vi "test_F9P_fgv-ver.vi"() -> ()   [LabVIEW 2019] (continued)
357,28,09,08,194,,1*72\r\n$GBGSV,5,3,17,10,14,222,31,11,34,144,33,13,50,316,32,14,73,036,27,1*77\r\n$GBGSV,5,4,17,16,25,186,,27,10,317,,28,61,308,30,33,75,244,42,1*7C\r\n$GBGSV,5,5,17,34,11,143,22,1*41\r\n$GBGSV,5,1,17,01,42,153,,03,45,207,,04,35,133,,05,09,257,,3*7E\r\n$GBGSV,5,2,17,06,29,183,,07,08,201,,08,66,357,16,09,08,194,,3*7D\r\n$GBGSV,5,3,17,10,14,222,32,11,34,144,46,13,50,316,21,14,73,036,27,3*76\r\n$GBGSV,5,4,17,16,25,186,36,27,10,317,,28,61,308,,33,75,244,,3*7E\r\n$GBGSV,5,5,17,34,11,143,,3*43\r\n$GNGLL,3723.57124,N,12657.01326,E,064943.00,A,A*7A\r\n$GNRMC,064944.00,A,3723.57121,N,12657.01327,E,0.019,,250720,,,A,V*10\r\n$GNVTG,,T,,M,0.019,N,0.036,K,A*30\r\n$GNGGA,064944.00,3723.57121,N,12657.01327,E,1,12,0.74,36.2,M,18.5,M,,*77\r\n$GNGSA,A,3,17,19,06,12,05,02,09,,,,,,1.35,0.74,1.12,1*02\r\n$GNGSA,A,3,85,70,71,72,,,,,,,,,1.35,0.74,1.12,2*0D\r\n$GNGSA,A,3,36,11,04,09,12,,,,,,,,1.35,0.74,1.12,3*0E\r\n$GNGSA,A,3,28,11,14,13,33,08,34,10,,,,,1.35,0.74,1.12,4*01\r\n$GPGSV,4,1,13,02,67,338,32,04,06,036,21,05,50,265,44,06,56,081,46,1*62\r\n$GPGSV,4,2,13,07,08,102,19,09,36,055,39,12,17,260,32,13,11,191,31,1*6B\r\n$GPGSV,4,3,13,17,16,158,42,19,34,162,41,25,11,291,25,29,09,322,35,1*68\r\n$GPGSV,4,4,13,30,03,132,,1*56\r\n$GPGSV,4,1,13,02,67,338,,04,06,036,,05,50,265,35,06,56,081,33,6*63\r\n$GPGSV,4,2,13,07,08,102,,09,36,055,22,12,17,260,30,13,11,191,,6*6E\r\n$GPGSV,4,3,13,17,16,158,35,19,34,162,,25,11,291,22,29,09,322,13,6*69\r\n$GPGSV,4,4,13,30,03,132,,6*51\r\n$GLGSV,2,1,06,70,51,030,19,71,72,230,44,72,20,218,35,84,06,136,08,1*7B\r\n$GLGSV,2,2,06,85,61,118,44,86,55,338,,1*7A\r\n$GLGSV,2,1,06,70,51,030,,71,72,230,28,72,20,218,36,84,06,136,13,3*72\r\n$GLGSV,2,2,06,85,61,118,33,86,55,338,,3*78\r\n$GAGSV,3,1,09,02,03,285,07,04,67,079,38,05,00,212,,09,47,197,33,7*70\r\n$GAGSV,3,2,09,11,78,050,29,12,30,117,32,18,58,277,45,19,15,041,08,7*7A\r\n$GAGSV,3,3,09,36,37,315,19,7*44\r\n$GAGSV,3,1,09,02,03,285,,04,67,079,29,05,00,212,,09,47,197,41,2*77\r\n$GAGSV,3,2,09,11,78,050,31,12,30,117,34,18,58,277,35,19,15,041,,2*7F\r\n$GAGSV,3,3,09,36,37,315,32,2*48\r\n$GBGSV,5,1,17,01,42,153,,03,45,207,,04,35,133,,05,09,257,,1*7C\r\n$GBGSV,5,2,17,06,29,183,,07,08,201,,08,66,357,29,09,08,194,,1*73\r\n$GBGSV,5,3,17,10,14,222,35,11,34,144,34,13,50,316,31,14,73,036,32,1*73\r\n$GBGSV,5,4,17,16,25,186,,27,10,317,,28,61,308,30,33,75,244,42,1*7C\r\n$GBGSV,5,5,17,34,11,143,23,1*40\r\n$GBGSV,5,1,17,01,42,153,,03,45,207,,04,35,133,,05,09,257,,3*7E\r\n$GBGSV,5,2,17,06,29,183,,07,08,201,,08,66,357,17,09,08,194,,3*7C\r\n$GBGSV,5,3,17,10,14,222,41,11,34,144,45,13,50,316,22,14,73,036,32,3*76\r\n$GBGSV,5,4,17,16,25,186,36,27,10,317,,28,61,308,,33,75,244,,3*7E\r\n$GBGSV,5,5,17,34,11,143,,3*43\r\n$GNGLL,3723.57121,N,12657.01327,E,064944.00,A,A*79\r\n$GNRMC,064945.00,A,3723.57119,N,12657.01328,E,0.031,,250720,,,A,V*1F\r\n$GNVTG,,T,,M,0.031,N,0.058,K,A*32\r\n$GNGGA,064945.00,3723.57119,N,12657.01328,E,1,12,0.74,36.2,M,18.5,M,,*72\r\n$GNGSA,A,3,17,19,06,12,05,02,09,,,,,,1.34,0.74,1.12,1*03\r\n$GNGSA,A,3,85,70,71,72,,,,,,,,,1.34,0.74,1.12,2*0C\r\n$GNGSA,A,3,36,11,04,09,12,,,,,,,,1.34,0.74,1.12,3*0F\r\n$GNGSA,A,3,28,11,14,13,33,08,34,10,,,,,1.34,0.74,1.12,4*00\r\n$GPGSV,4,1,13,02,67,338,34,04,06,036,21,05,50,265,44,06,56,081,46,1*64\r\n$GPGSV,4,2,13,07,08,102,18,09,36,055,39,12,17,260,31,13,11,191,32,1*6A\r\n$GPGSV,4,3,13,17,16,158,43,19,34,162,41,25,11,291,24,29,09,322,35,1*68\r\n$GPGSV,4,4,13,30,03,132,,1*56\r\n$GPGSV,4,1,13,02,67,338,,04,06,036,,05,50,265,33,06,56,081,34,6*62\r\n$GPGSV,4,2,13,07,08,102,,09,36,055,22,12,17,260,21,13,11,191,,6*6E\r\n$GPGSV,4,3,13,17,16,158,34,19,34,162,,25,11,291,24,29,09,322,13,6*6E\r\n$GPGSV,4,4,13,30,03,132,,6*51\r\n$GLGSV,2,1,06,70,51,030,18,71,72,230,44,72,20,218,35,84,06,136,09,1*7B\r\n$GLGSV,2,2,06,85,61,118,45,86,55,338,,1*7B\r\n$GLGSV,2,1,06,70,51,030,,71,72,230,29,72,20,218,36,84,06,136,16,3*76\r\n$GLGSV,2,2,06,85,61,118,33,86,55,338,,3*78\r\n$GAGSV,3,1,09,02,03,285,09,04,67,079,37,05,00,212,,09,47,197,32,7*70\r\n$GAGSV,3,2,09,11,78,050,31,12,30,117,33,18,58,277,45,19,15,041,08,7*72\r\n$GAGSV,3,3,09,36,37,315,22,7*4C\r\n$GAGSV,3,1,09,02,03,285,,04,67,079,30,05,00,212,,09,47,197,41,2*7F\r\n$GAGSV,3,2,09,11,78,050,31,12,30,117,33,18,58,277,35,19,15,041,,2*78\r\n$GAGSV,3,3,09,36,37,315,30,2*4A\r\n$GBGSV,5,1,17,01,42,153,,03,45,207,,04,35,133,,05,09,257,,1*7C\r\n$GBGSV,5,2,17,06,29,183,,07,08,201,,08,66,357,28,09,08,194,,1*72\r\n$GBGSV,5,3,17,10,14,222,35,11,34,144,35,13,50,316,32,14,73,036,32,1*71\r\n$GBGSV,5,4,17,16,25,186,,27,10,317,,28,61,308,32,33,75,244,42,1*7E\r\n$GBGSV,5,5,17,34,11,143,23,1*40\r\n$GBGSV,5,1,17,01,42,153,,03,45,207,,04,35,133,,05,09,257,,3*7E\r\n$GBGSV,5,2,17,06,29,183,,07,08,201,,08,66,357,16,09,08,194,,3*7D\r\n$GBGSV,5,3,17,10,14,222,38,11,34,144,45,13,50,316,21,14,73,036,32,3*7B\r\n$GBGSV,5,4,17,16,25,186,35,27,10,317,,28,61,308,,33,75,244,,3*7D\r\n$GBGSV,5,5,17,34,11,143,,3*43\r\n$GNGLL,3723.57119,N,12657.01328,E,064945.00,A,A*7C\r\n$GNRMC,064946.00,A,3723.57118,N,12657.01329,E,0.032,,250720,,,A,V*1F\r\n$GNVTG,,T,,M,0.032,N,0.059,K,A*30\r\n$GNGGA,064946.00,3723.57118,N,12657.01329,E,1,12,0.65,36.1,M,18.5,M,,*72\r\n$GNGSA,A,3,17,19,06,12,05,02,09,,,,,,1.11,0.65,0.90,1*0F\r\n$GNGSA,A,3,85,70,71,72,,,,,,,,,1.11,0.65,0.90,2*00\r\n$GNGSA,A,3,36,19,11,04,09,12,,,,,,,1.11,0.65,0.90,3*0B\r\n$GNGSA,A,3,28,11,14,13,33,08,34,10,,,,,1.11,0.65,0.90,4*0C\r\n$GPGSV,4,1,13,02,67,338,34,04,06,036,20,05,50,265,44,06,56,081,45,1*66\r\n$GPGSV,4,2,13,07,08,102,,09,36,055,40,12,17,260,32,13,11,191,30,1*6C\r\n$GPGSV,4,3,13,17,16,158,43,19,34,162,41,25,11,291,23,29,09,322,35,1*6F\r\n$GPGSV,4,4,13,30,03,132,,1*56\r\n$GPGSV,4,1,13,02,67,338,,04,06,036,,05,50,265,32,06,56,081,35,6*62\r\n$GPGSV,4,2,13,07,08,102,,09,36,055,22,12,17,260,20,13,11,191,,6*6F\r\n$GPGSV,4,3,13,17,16,158,34,19,34,162,,25,11,291,25,29,09,322,13,6*6F\r\n$GPGSV,4,4,13,30,03,132,,6*51\r\n$GLGSV,2,1,06,70,51,030,15,71,72,230,44,72,20,218,35,84,06,136,09,1*76\r\n$GLGSV,2,2,06,85,61,118,45,86,55,338,,1*7B\r\n$GLGSV,2,1,06,70,51,030,,71,72,230,30,72,20,218,36,84,06,136,13,3*7B\r\n$GLGSV,2,2,06,85,61,118,33,86,55,338,,3*78\r\n$GAGSV,3,1,09,02,03,285,08,04,67,079,36,05,00,212,,09,47,197,32,7*70\r\n$GAGSV,3,2,09,11,78,050,31,12,30,117,33,18,58,277,45,19,15,041,11,7*7A\r\n$GAGSV,3,3,09,36,37,315,23,7*4D\r\n$GAGSV,3,1,09,02,03,285,,04,67,079,30,05,00,212,,09,47,197,41,2*7F\r\n$GAGSV,3,2,09,11,78,050,30,12,30,117,33,18,58,277,34,19,15,041,,2*78\r\n$GAGSV,3,3,09,36,37,315,30,2*4A\r\n$GBGSV,5,1,17,01,42,153,,03,45,207,,04,35,133,,05,09,257,,1*7C\r\n$GBGSV,5,2,17,06,29,183,,07,08,201,,08,66,357,27,09,08,194,,1*7D\r\n$GBGSV,5,3,17,10,14,222,35,11,34,144,35,13,50,316,32,14,73,036,33,1*70\r\n$GBGSV,5,4,17,16,25,186,,27,10,317,,28,61,308,32,33,75,244,43,1*7F\r\n$GBGSV,5,5,17,34,11,143,24,1*47\r\n$GBGSV,5,1,17,01,42,153,,03,45,207,,04,35,133,,05,09,257,,3*7E\r\n$GBGSV,5,2,17,06,29,183,,07,08,201,,08,66,357,14,09,08,194,,3*7F\r\n$GBGSV,5,3,17,10,14,222,38,11,34,144,45,13,50,316,21,14,73,036,32,3*7B\r\n$GBGSV,5,4,17,16,25,186,36,27,10,317,,28,61,308,,33,75,244,,3*7E\r\n$GBGSV,5,5,17,34,11,143,,3*43\r\n$GNGLL,3723.57118,N,12657.01329,E,064946.00,A,A*7F\r\n$GNRMC,064947.00,A,3723.57116,N,12657.01329,E,0.035,,250720,,,A,V*17\r\n$GNVTG,,T,,M,0.035,N,0.065,K,A*38\r\n$GNGGA,064947.00,3723.57116,N,12657.01329,E,1,12,0.65,36.1,M,18.5,M,,*7D\r\n$GNGSA,A,3,17,19,06,12,05,02,09,,,,,,1.11,0.65,0.90,1*0F\r\n$GNGSA,A,3,85,70,71,72,,,,,,,,,1.11,0.65,0.90,2*00\r\n$GNGSA,A,3,36,19,11,04,09,12,,,,,,,1.11,0.65,0.90,3*0B\r\n$GNGSA,A,3,28,11,14,13,33,08,34,10,,,,,1.11,0.65,0.90,4*0C\r\n$GPGSV,4,1,13,02,67,338,33,04,06,036,19,05,50,265,43,06,56,081,44,1*6D\r\n$GPGSV,4,2,13,07,08,102,22,09,36,055,40,12,17,260,32,13,11,191,29,1*64\r\n$GPGSV,4,3,13,17,16,158,43,19,34,162,42,25,11,291,20,29,09,322,35,1*6F\r\n$GPGSV,4,4,13,30,03,132,,1*56\r\n$GPGSV,4,1,13,02,67,338,,04,06,036,,05,50,265,32,06,56,081,35,6*62\r\n$GPGSV,4,2,13,07,08,102,,09,36,055,23,12,17,260,18,13,11,191,,6*65\r\n$GPGSV,4,3,13,17,16,158,34,19,34,162,,25,11,291,25,29,09,322,12,6*6E\r\n$GPGSV,4,4,13,30,03,132,,6*51\r\n$GLGSV,2,1,06,70,51,030,14,71,72,230,45,72,20,218,34,84,06,136,09,1*77\r\n$GLGSV,2,2,06,85,61,118,45,86,55,338,,1*7B\r\n$GLGSV,2,1,06,70,51,030,,71,72,230,29,72,20,218,34,84,06,136,13,3*71\r\n$GLGSV,2,2,06,85,61,118,31,86,55,338,,3*7A\r\n$GAGSV,3,1,09,02,03,285,09,04,67,079,36,05,00,212,,09,47,197,31,7*72\r\n$GAGSV,3,2,09,11,78,050,30,12,30,117,35,18,58,277,45,19,15,041,14,7*78\r\n$GAGSV,3,3,09,36,37,315,24,7*4A\r\n$GAGSV,3,1,09,02,03,285,,04,67,079,30,05,00,212,,09,47,197,41,2*7F\r\n$GAGSV,3,2,09,11,78,050,31,12,30,117,33,18,58,277,34,19,15,041,,2*79\r\n$GAGSV,3,3,09,36,37,315,30,2*4A\r\n$GBGSV,5,1,17,01,42,153,,03,45,207,,04,35,133,,05,09,257,,1*7C\r\n$GBGSV,5,2,17,06,29,183,,07,08,201,,08,66,357,27,09,08,194,,1*7D\r\n$GBGSV,5,3,17,10,14,222,35,11,34,144,35,13,50,316,31,14,73,036,33,1*73\r\n$GBGSV,5,4,17,16,25,186,,27,10,317,,28,61,308,32,33,75,244,43,1*7F\r\n$GBGSV,5,5,17,34,11,143,24,1*47\r\n$GBGSV,5,1,17,01,42,153,,03,45,207,,04,35,133,,05,09,257,,3*7E\r\n$GBGSV,5,2,17,06,29,183,,07,08,201,,08,66,357,10,09,08,194,,3*7B\r\n$GBGSV,5,3,17,10,14,222,39,11,34,144,45,13,50,316,22,14,73,036,32,3*79\r\n$GBGSV,5,4,17,16,25,186,36,27,10,317,,28,61,308,,33,75,244,,3*7E\r\n$GBGSV,5,5,17,34,11,143,,3*43\r\n$GNGLL,3723.57116,N,12657.01329,E,064947.00,A,A*70\r\n$GNRMC,064948.00,A,3723.57114,N,12657.01331,E,0.061,,250720,,,A,V*12\r\n$GNVTG,,T,,M,0.061,N,0.112,K,A*38\r\n$GNGGA,064948.00,3723.57114,N,12657.01331,E,1,12,0.62,36.1,M,18.5,M,,*7E\r\n$GNGSA,A,3,17,19,06,12,05,02,09,,,,,,1.04,0.62,0.84,1*09\r\n$GNGSA,A,3,85,70,71,72,,,,,,,,,1.04,0.62,0.84,2*06\r\n$GNGSA,A,3,36,19,11,04,09,12,,,,,,,1.04,0.62,0.84,3*0D\r\n$GNGSA,A,3,28,11,14,13,33,08,34,10,,,,,1.04,0.62,0.84,4*0A\r\n$GPGSV,4,1,13,02,67,338,33,04,06,036,18,05,50,265,44,06,56,081,45,1*6A\r\n$GPGSV,4,2,13,07,08,102,20,09,36,055,40,12,17,260,30,13,11,191,29,1*64\r\n$GPGSV,4,3,13,17,16,158,43,19,34,162,42,25,11,291,21,29,09,322,35,1*6E\r\n$GPGSV,4,4,13,30,03,132,,1*56\r\n$GPGSV,4,1,13,02,67,338,,04,06,036,,05,50,265,32,06,56,081,35,6*62\r\n$GPGSV,4,2,13,07,08,102,,09,36,055,26,12,17,260,20,13,11,191,,6*6B\r\n$GPGSV,4,3,13,17,16,158,34,19,34,162,,25,11,291,25,29,09,322,11,6*6D\r\n$GPGSV,4,4,13,30,03,132,,6*51\r\n$GLGSV,2,1,06,70,51,030,16,71,72,230,44,72,20,218,31,84,06,136,11,1*78\r\n$GLGSV,2,2,06,85,61,118,45,86,55,338,,1*7B\r\n$GLGSV,2,1,06,70,51,030,,71,72,230,29,72,20,218,36,84,06,136,15,3*75\r\n$GLGSV,2,2,06,85,61,118,32,86,55,338,,3*79\r\n$GAGSV,3,1,09,02,03,285,07,04,67,079,37,05,00,212,,09,47,197,31,7*7D\r\n$GAGSV,3,2,09,11,78,050,30,12,30,117,33,18,58,277,46,19,15,041,14,7*7D\r\n$GAGSV,3,3,09,36,37,315,25,7*4B\r\n$GAGSV,3,1,09,02,03,285,,04,67,079,30,05,00,212,,09,47,197,41,2*7F\r\n$GAGSV,3,2,09,11,78,050,30,12,30,117,33,18,58,277,34,19,15,041,,2*78\r\n$GAGSV,3,3,09,36,37,315,30,2*4A\r\n$GBGSV,5,1,17,01,42,153,,03,45,207,,04,35,133,,05,09,257,,1*7C\r\n$GBGSV,5,2,17,06,29,183,,07,08,201,,08,66,357,27,09,08,194,,1*7D\r\n$GBGSV,5,3,17,10,14,222,35,11,34,144,34,13,50,316,31,14,73,036,32,1*73\r\n$GBGSV,5,4,17,16,25,186,,27,10,317,,28,61,308,33,33,75,244,43,1*7E\r\n$GBGSV,5,5,17,34,11,143,23,1*40\r\n$GBGSV,5,1,17,01,42,153,,03,45,207,,04,35,133,,05,09,257,,3*7E\r\n$GBGSV,5,2,17,06,29,183,,07,08,201,,08,66,357,12,09,08,194,,3*79\r\n$GBGSV,5,3,17,10,14,222,38,11,34,144,45,13,50,316,22,14,73,036,32,3*78\r\n$GBGSV,5,4,17,16,25,186,36,27,10,317,,28,61,308,,33,75,244,,3*7E\r\n$GBGSV,5,5,17,34,11,143,,3*43\r\n$GNGLL,3723.57114,N,12657.01331,E,064948.00,A,A*74\r\n$GNRMC,064949.00,A,3723.57112,N,12657.01332,E,0.017,,250720,,,A,V*17\r\n$GNVTG,,T,,M,0.017,N,0.031,K,A*39\r\n$GNGGA,064949.00,3723.57112,N,12657.01332,E,1,12,0.62,36.1,M,18.5,M,,*7A\r\n$GNGSA,A,3,17,19,06,12,05,02,09,,,,,,1.04,0.62,0.84,1*09\r\n$GNGSA,A,3,85,70,71,72,,,,,,,,,1.04,0.62,0.84,2*06\r\n$GNGSA,A,3,36,19,11,04,09,12,,,,,,,1.04,0.62,0.84,3*0D\r\n$GNGSA,A,3,28,11,14,13,33,08,34,10,,,,,1.04,0.62,0.84,4*0A\r\n$GPGSV,4,1,13,02,67,338,32,04,06,036,17,05,50,265,44,06,56,081,45,1*64\r\n$GPGSV,4,2,13,07,08,102,,09,36,055,38,12,17,260,31,13,11,191,30,1*60\r\n$GPGSV,4,3,13,17,16,158,43,19,34,162,42,25,11,291,20,29,09,322,35,1*6F\r\n$GPGSV,4,4,13,30,03,132,,1*56\r\n$GPGSV,4,1,13,02,67,338,,04,06,036,,05,50,265,32,06,56,081,34,6*63\r\n$GPGSV,4,2,13,07,08,102,,09,36,055,26,12,17,260,19,13,11,191,,6*61\r\n$GPGSV,4,3,13,17,16,158,34,19,34,162,,25,11,291,25,29,09,322,,6*6D\r\n$GPGSV,4,4,13,30,03,132,,6*51\r\n$GLGSV,2,1,06,70,51,030,17,71,72,230,45,72,20,218,35,84,06,136,10,1*7D\r\n$GLGSV,2,2,06,85,61,118,45,86,55,338,,1*7B\r\n$GLGSV,2,1,06,70,51,030,,71,72,230,30,72,20,218,36,84,06,136,10,3*78\r\n$GLGSV,2,2,06,85,61,118,33,86,55,338,,3*78\r\n$GAGSV,3,1,09,02,03,285,11,04,67,079,37,05,00,212,,09,47,197,30,7*7B\r\n$GAGSV,3,2,09,11,78,050,30,12,30,117,33,18,58,277,46,19,15,041,14,7*7D\r\n$GAGSV,3,3,09,36,37,315,24,7*4A\r\n$GAGSV,3,1,09,02,03,285,,04,67,079,30,05,00,212,,09,47,197,41,2*7F\r\n$GAGSV,3,2,09,11,78,050,30,12,30,117,32,18,58,277,34,19,15,041,,2*79\r\n$GAGSV,3,3,09,36,37,315,29,2*42\r\n$GBGSV,5,1,17,01,42,153,,03,45,207,,04,35,133,,05,09,257,,1*7C\r\n$GBGSV,5,2,17,06,29,183,,07,08,201,,08,66,357,26,09,08,194,,1*7C\r\n$GBGSV,5,3,17,10,14,222,35,11,34,144,34,13,50,316,33,14,73,036,32,1*71\r\n$GBGSV,5,4,17,16,25,186,,27,10,317,,28,61,308,33,33,75,244,43,1*7E\r\n$GBGSV,5,5,17,34,11,143,23,1*40\r\n$GBGSV,5,1,17,01,42,153,,03,45,207,,04,35,133,,05,09,257,,3*7E\r\n$GBGSV,5,2,17,06,29,183,,07,08,201,,08,66,357,,09,08,194,,3*7A\r\n$GBGSV,5,3,17,10,14,222,38,11,34,144,45,13,50,316,21,14,73,036,32,3*7B\r\n$GBGSV,5,4,17,16,25,186,36,27,10,317,,28,61,308,,33,75,244,,3*7E\r\n$GBGSV,5,5,17,34,11,143,,3*43\r\n$GNGLL,3723.57112,N,12657.01332,E,064949.00,A,A*70\r\n$GNRMC,064950.00,A,3723.57110,N,12657.01333,E,0.004,,250720,,,A,V*1E\r\n$GNVTG,,T,,M,0.004,N,0.007,K,A*3E\r\n$GNGGA,064950.00,3723.57110,N,12657.01333,E,1,12,0.65,36.1,M,18.5,M,,*76\r\n$GNGSA,A,3,17,19,06,12,05,02,09,,,,,,1.11,0.65,0.90,1*0F\r\n$GNGSA,A,3,85,70,71,72,,,,,,,,,1.11,0.65,0.90,2*00\r\n$GNGSA,A,3,36,19,11,04,09,12,,,,,,,1.11,0.65,0.90,3*0B\r\n$GNGSA,A,3,28,11,14,13,33,08,34,10,,,,,1.11,0.65,0.90,4*0C\r\n$GPGSV,4,1,13,02,67,338,32,04,06,036,15,05,50,265,44,06,56,081,46,1*65\r\n$GPGSV,4,2,13,07,08,102,19,09,36,055,39,12,17,260,37,13,11,191,30,1*6F\r\n$GPGSV,4,3,13,17,16,158,44,19,34,162,42,25,11,291,21,29,09,322,24,1*69\r\n$GPGSV,4,4,13,30,03,132,,1*56\r\n$GPGSV,4,1,13,02,67,338,,04,06,036,,05,50,265,31,06,56,081,35,6*61\r\n$GPGSV,4,2,13,07,08,102,,09,36,055,26,12,17,260,18,13,11,191,,6*60\r\n$GPGSV,4,3,13,17,16,158,34,19,34,162,,25,11,291,25,29,09,322,,6*6D\r\n$GPGSV,4,4,13,30,03,132,,6*51\r\n$GLGSV,2,1,06,70,51,030,19,71,72,230,45,72,20,218,35,84,06,136,11,1*72\r\n$GLGSV,2,2,06,85,61,118,45,86,55,338,,1*7B\r\n$GLGSV,2,1,06,70,51,030,,71,72,230,30,72,20,218,37,84,06,136,13,3*7A\r\n$GLGSV,2,2,06,85,61,118,33,86,55,338,,3*78\r\n$GAGSV,3,1,09,02,03,285,08,04,67,079,38,05,00,212,,09,47,197,30,7*7C\r\n$GAGSV,3,2,09,11,78,050,31,12,30,117,32,18,58,277,46,19,15,041,14,7*7D\r\n$GAGSV,3,3,09,36,37,315,23,7*4D\r\n$GAGSV,3,1,09,02,03,285,,04,67,079,29,05,00,212,,09,47,197,41,2*77\r\n$GAGSV,3,2,09,11,78,050,30,12,30,117,33,18,58,277,34,19,15,041,,2*78\r\n$GAGSV,3,3,09,36,37,315,29,2*42\r\n$GBGSV,5,1,17,01,42,153,,03,45,207,,04,35,133,,05,09,257,,1*7C\r\n$GBGSV,5,2,17,06,29,183,,07,08,201,,08,66,357,28,09,08,194,,1*72\r\n$GBGSV,5,3,17,10,14,222,35,11,34,144,35,13,50,316,33,14,73,036,33,1*71\r\n$GBGSV,5,4,17,16,25,186,,27,10,317,,28,61,307,33,33,75,244,43,1*71\r\n$GBGSV,5,5,17,34,11,143,22,1*41\r\n$GBGSV,5,1,17,01,42,153,,03,45,207,,04,35,133,,05,09,257,,3*7E\r\n$GBGSV,5,2,17,06,29,183,,07,08,201,,08,66,357,,09,08,194,,3*7A\r\n$GBGSV,5,3,17,10,14,222,38,11,34,144,46,13,50,316,23,14,73,036,33,3*7B\r\n$GBGSV,5,4,17,16,25,186,36,27,10,317,,28,61,307,,33,75,244,,3*71\r\n$GBGSV,5,5,17,34,11,143,,3*43\r\n$GNGLL,3723.57110,N,12657.01333,E,064950.00,A,A*7B\r\n$GNRMC,064951.00,A,3723.57107,N,12657.01334,E,0.013,,250720,,,A,V*18\r\n$GNVTG,,T,,M,0.013,N,0.024,K,A*39\r\n$GNGGA,064951.00,3723.57107,N,12657.01334,E,1,12,0.65,36.0,M,18.5,M,,*77\r\n$GNGSA,A,3,17,19,06,12,05,02,09,,,,,,1.11,0.65,0.90,1*0F\r\n$GNGSA,A,3,85,70,71,72,,,,,,,,,1.11,0.65,0.90,2*00\r\n$GNGSA,A,3,36,19,11,04,09,12,,,,,,,1.11,0.65,0.90,3*0B\r\n$GNGSA,A,3,28,11,14,13,33,08,34,10,,,,,1.11,0.65,0.90,4*0C\r\n$GPGSV,4,1,13,02,67,338,37,04,06,036,13,05,50,265,43,06,56,081,45,1*62\r\n$GPGSV,4,2,13,07,08,102,,09,36,055,39,12,17,260,28,13,11,191,31,1*68\r\n$GPGSV,4,3,13,17,16,158,43,19,34,162,42,25,11,291,20,29,09,322,23,1*68\r\n$GPGSV,4,4,13,30,03,132,,1*56\r\n$GPGSV,4,1,13,02,67,338,,04,06,036,,05,50,265,31,06,56,081,35,6*61\r\n$GPGSV,4,2,13,07,08,102,,09,36,055,26,12,17,260,16,13,11,191,,6*6E\r\n$GPGSV,4,3,13,17,16,158,34,19,34,162,,25,11,291,26,29,09,322,,6*6E\r\n$GPGSV,4,4,13,30,03,132,,6*51\r\n$GLGSV,2,1,06,70,51,030,18,71,72,230,44,72,20,218,31,84,06,136,08,1*7E\r\n$GLGSV,2,2,06,85,61,118,44,86,55,338,,1*7A\r\n$GLGSV,2,1,06,70,51,030,,71,72,230,29,72,20,218,36,84,06,136,11,3*71\r\n$GLGSV,2,2,06,85,61,118,32,86,55,338,,3*79\r\n$GAGSV,3,1,09,02,03,285,10,04,67,079,39,05,00,212,,09,47,197,31,7*75\r\n$GAGSV,3,2,09,11,78,050,32,12,30,117,33,18,58,277,46,19,15,041,14,7*7F\r\n$GAGSV,3,3,09,36,37,315,25,7*4B\r\n$GAGSV,3,1,09,02,03,285,,04,67,079,30,05,00,212,,09,47,197,41,2*7F\r\n$GAGSV,3,2,09,11,78,050,30,12,30,117,33,18,58,277,34,19,15,041,,2*78\r\n$GAGSV,3,3,09,36,37,315,29,2*42\r\n$GBGSV,5,1,17,01,42,153,,03,45,207,,04,35,133,,05,09,257,,1*7C\r\n$GBGSV,5,2,17,06,29,183,,07,08,201,,08,66,357,28,09,08,194,,1*72\r\n$GBGSV,5,3,17,10,14,222,35,11,34,144,36,13,50,316,33,14,73,036,35,1*74\r\n$GBGSV,5,4,17,16,25,186,,27,10,317,,28,61,307,34,33,75,244,43,1*76\r\n$GBGSV,5,5,17,34,11,143,20,1*43\r\n$GBGSV,5,1,17,01,42,153,,03,45,207,,04,35,133,,05,09,257,,3*7E\r\n$GBGSV,5,2,17,06,29,183,,07,08,201,,08,66,357,,09,08,194,,3*7A\r\n$GBGSV,5,3,17,10,14,222,36,11,34,144,45,13,50,316,22,14,73,036,32,3*76\r\n$GBGSV,5,4,17,16,25,186,36,27,10,317,,28,61,307,,33,75,244,,3*71\r\n$GBGSV,5,5,17,34,11,143,,3*43\r\n$GNGLL,3723.57107,N,12657.01334,E,064951.00,A,A*7B\r\n$GNRMC,064952.00,A,3723.57105,N,12657.01334,E,0.038,,250720,,,A,V*10\r\n$GNVTG,,T,,M,0.038,N,0.070,K,A*31\r\n$GNGGA,064952.00,3723.57105,N,12657.01334,E,1,12,0.65,36.0,M,18.5,M,,*76\r\n$GNGSA,A,3,17,19,06,12,05,02,09,,,,,,1.11,0.65,0.90,1*0F\r\n$GNGSA,A,3,85,70,71,72,,,,,,,,,1.11,0.65,0.90,2*00\r\n$GNGSA,A,3,36,19,11,04,09,12,,,,,,,1.11,0.65,0.90,3*0B\r\n$GNGSA,A,3,28,11,14,13,33,08,34,10,,,,,1.11,0.65,0.90,4*0C\r\n$GPGSV,4,1,13,02,67,338,33,04,06,036,12,05,50,265,43,06,56,081,47,1*65\r\n$GPGSV,4,2,13,07,08,102,,09,36,055,41,12,17,260,27,13,11,191,30,1*69\r\n$GPGSV,4,3,13,17,16,158,44,19,34,162,43,25,11,291,19,29,09,322,,1*65\r\n$GPGSV,4,4,13,30,03,132,,1*56\r\n$GPGSV,4,1,13,02,67,338,,04,06,036,,05,50,265,31,06,56,081,36,6*62\r\n$GPGSV,4,2,13,07,08,102,,09,36,055,26,12,17,260,18,13,11,191,,6*60\r\n$GPGSV,4,3,13,17,16,158,34,19,34,162,,25,11,291,26,29,09,322,,6*6E\r\n$GPGSV,4,4,13,30,03,132,,6*51\r\n$GLGSV,2,1,06,70,51,030,17,71,72,230,44,72,20,218,31,84,06,136,10,1*78\r\n$GLGSV,2,2,06,85,61,118,44,86,55,338,,1*7A\r\n$GLGSV,2,1,06,70,51,030,,71,72,230,29,72,20,218,35,84,06,136,11,3*72\r\n$GLGSV,2,2,06,85,61,118,32,86,55,338,,3*79\r\n$GAGSV,3,1,09,02,03,285,09,04,67,079,38,05,00,212,,09,47,197,30,7*7D\r\n$GAGSV,3,2,09,11,78,050,31,12,30,117,33,18,58,277,46,19,15,041,13,7*7B\r\n$GAGSV,3,3,09,36,37,315,23,7*4D\r\n$GAGSV,3,1,09,02,03,285,,04,67,079,29,05,00,212,,09,47,197,41,2*77\r\n$GAGSV,3,2,09,11,78,050,30,12,30,117,33,18,58,277,34,19,15,041,,2*78\r\n$GAGSV,3,3,09,36,37,315,28,2*43\r\n$GBGSV,5,1,17,01,42,153,,03,45,207,,04,35,133,,05,09,257,,1*7C\r\n$GBGSV,5,2,17,06,29,183,,07,08,201,,08,66,357,28,09,08,194,,1*72\r\n$GBGSV,5,3,17,10,14,222,35,11,34,144,34,13,50,316,32,14,73,036,31,1*73\r\n$GBGSV,5,4,17,16,25,186,,27,10,317,,28,61,307,33,33,75,244,43,1*71\r\n$GBGSV,5,5,17,34,11,143,17,1*47\r\n$GBGSV,5,1,17,01,42,153,,03,45,207,,04,35,133,,05,09,257,,3*7E\r\n$GBGSV,5,2,17,06,29,183,,07,08,201,,
